vi "Test Descending Test Case Static Test Method.vi"(8 "error in (no error)":errorcluster, 11 "Descending Test Test Case in":refnum<class "Descending Test Test Case.lvclass">) -> (0 "error out":errorcluster, 3 "Descending Test Test Case out":refnum<class "Descending Test Test Case.lvclass">)   [LabVIEW 2020, in "Descending Test Test Case.lvclass"]
uses:
  Descending Test Test Case.lvclass
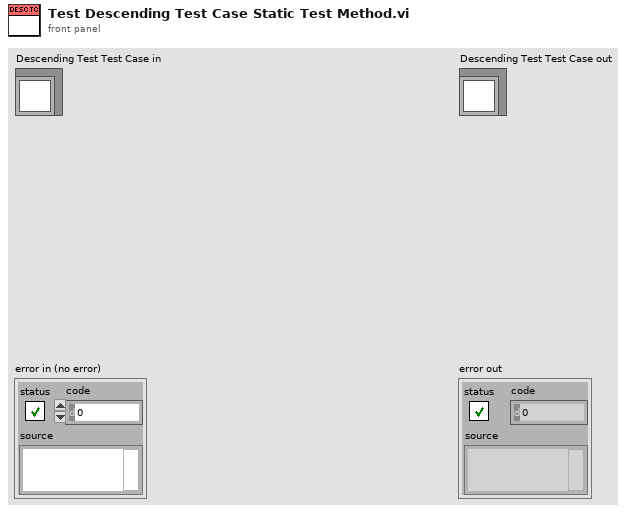
[diagram p1: front panel]
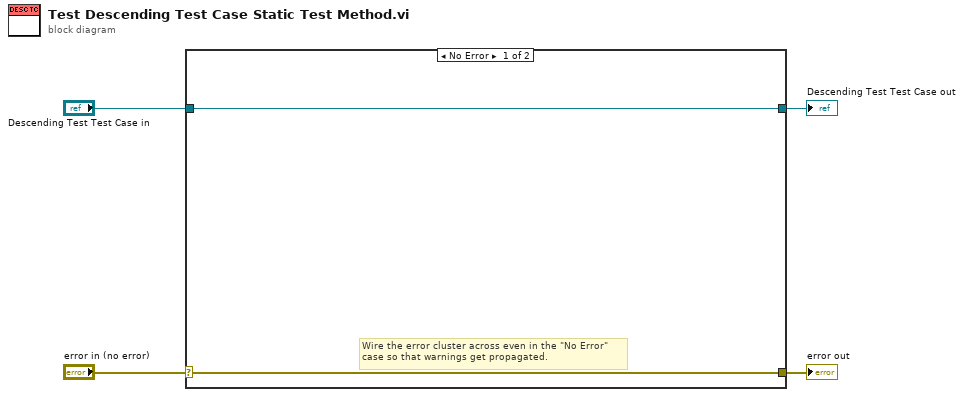
[diagram p0: block diagram]
diagram:
  n1 = case shown="No Error" "error in (no error)" {
    selector: "error in (no error)" -> [w5 w8]
    tunnel: [w5 w8] -> w3
    tunnel: [w6 w7] -> w1
    tunnel: "Descending Test Test Case in" -> [w6 w7]
    frame No Error {
      # "Wire the error cluster across even in the \"No Error\"\ncase so that warnings get propagated."
    }
    frame Error {
    }
  }
  "error out" <- w3
  "Descending Test Test Case out" <- w1
